vi "Array.vi"() -> ()   [LabVIEW 2020]
panel:
  out "Waveform Graph":dbl[][](graph)
  in  "Array":dbl[][](array[numeric])
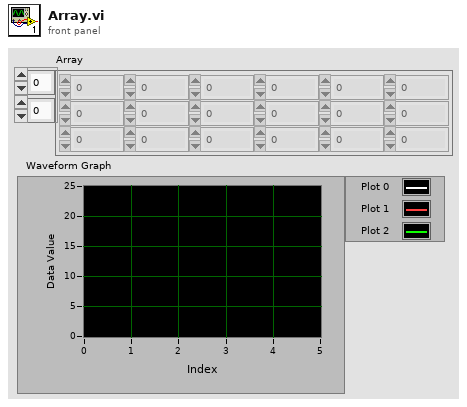
[diagram p1: front panel]
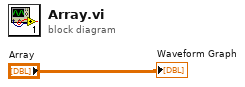
[diagram p0: block diagram]
diagram:
  "Waveform Graph" <- "Array"
